vi "Publish Build Progress.vi"(8 "error in (no error)":errorcluster, 9 "Total Number of Builds":dbl, 10 "Current Iteration":dbl, 11 "CD Build Tools in":refnum<class "Project Build Tools.lvclass">) -> (0 "error out":errorcluster, 3 "CD Build Tools out":refnum<class "Project Build Tools.lvclass">)   [LabVIEW 2019, in "Project Build Tools.lvclass"]
uses:
  Project Build Tools.lvclass
  Project Build Tools.lvclass/Project Build Tools.ctl
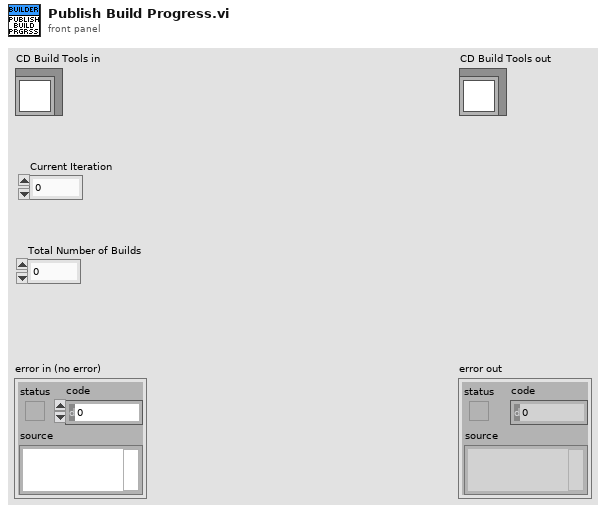
[diagram p1: front panel]
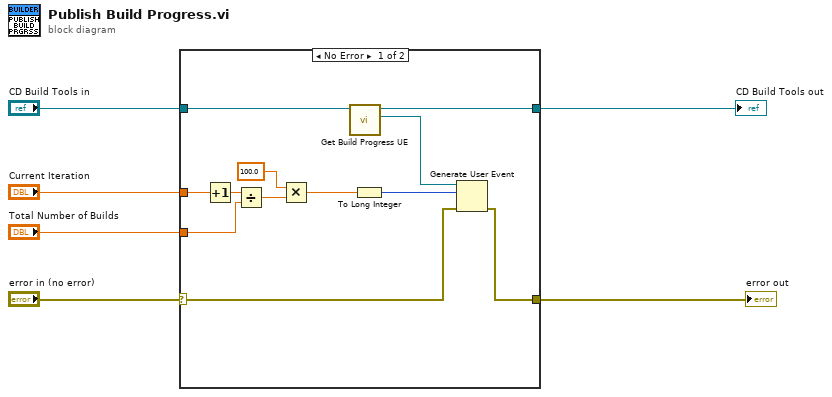
[diagram p0: block diagram]
diagram:
  n1 = case shown="No Error" "error in (no error)" {
    selector: "error in (no error)" -> [w10 w20]
    tunnel: [w9 w20] -> w5
    tunnel: [w12 w19] -> w3
    tunnel: "CD Build Tools in" -> [w13 w19]
    tunnel: "Total Number of Builds" -> [w8 _]
    tunnel: "Current Iteration" -> [w7 _]
    frame No Error {
      n2 = Increment(x=w7) -> (x+1=w14:dbl)
      n3 = Divide(x=w14, y=w8) -> (x/y=w18:dbl)
      n4 = Multiply(x=100.0, y=w18) -> (x*y=w16:dbl)
      n5 = call "Get Build Progress UE.vi"("CD Build Tools in"=w13) -> ("Build Progress UE"=w11:refnum<user-event>, "CD Build Tools out"=w12:refnum<class "Project Build Tools.lvclass">)  [unwired: 9 in]
      n6 = To Long Integer(number=w16) -> (32bit integer=w15:i32)
      n7 = Generate User Event(user event=w11, event data cluster=w15, error in=w10) -> (error out=w9:errorcluster)  [unwired: 1 in, 1 out]
    }
    frame Error {
    }
  }
  "error out" <- w5
  "CD Build Tools out" <- w3
